vi "Datacluster remove duplicates_sort_test.vi"(5 "Remove duplicate":bool=TRUE, 6 "tolerance":dbl format="%.3e", 7 "ascending":bool=TRUE, 9 "Sort?":bool=TRUE) -> ()   [LabVIEW 2020]
panel:
  out "comparative":dbl
  out "output":dbl[][](array[numeric])=[[0.0, 0.0, -1.0], [1.0, 3.0, 4.0], [2.0, 0.0, 0.0], [3.0, 0.0, 0.0], [4.0, 1.0, 0.0], [6.0, 0.0, 5.0], [7.0, 0.0, 0.0], [8.0, 0.0, 0.0], [9.0, 0.0, 0.0]]
  in  "all rows":dbl[][](array[numeric])=[[7.0, 0.0, 0.0], [0.0, 0.0, -1.0], [2.0, 0.0, 0.0], [4.0, 1.0, 0.0], [6.0, 0.0, 5.0], [7.0, 0.0, 0.0], [0.0, 0.0, 0.0], [1.0, 3.0, 4.0], [9.0, 0.0, 0.0], [2.0, 0.0, 0.0], [3.0, 0.0, 0.0], [0.0, 0.0, 0.0], [2.0, 0.0, 0.0], [8.0, 0.0, 0.0]]
  in  "target column":u16
  # "(1) Data are sorted ascending or descending order.\n(2) Remove duplicate\n      i) Neighboring two data points are compared, if determined to be a duplicate, the second data point will be removed.\n      ii) Repeat i) unitl no duplicates found."
  # "Caution: All rows will be affected."
  # "(1) Select datasets to be processed"
  # "(2) Sort"
  # "i) Sort ?"
  # "ii) Ascending or descendingwhich order?"
  # "descending"
  # "(3) Remove duplicate? Tolerance?"
  # "(duplicate if \ndata difference <= (max-min) * tolerance"
  # "(4) Start processing"
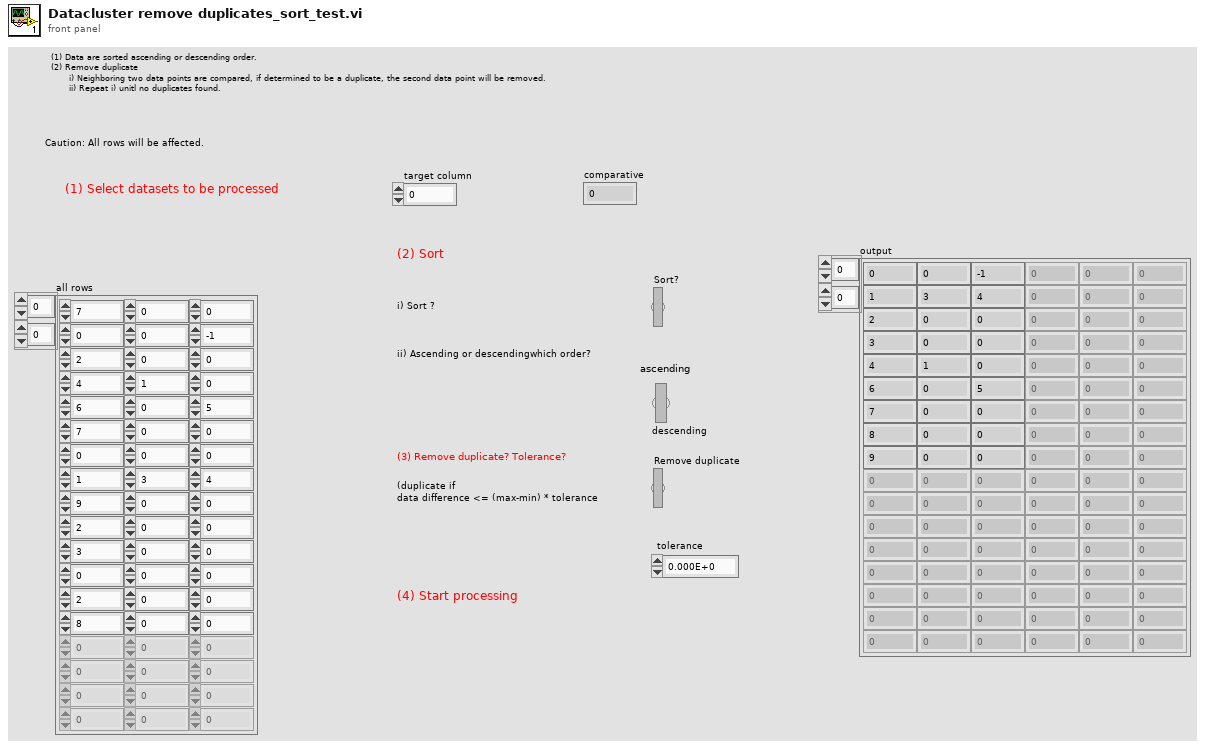
[diagram p1: front panel]
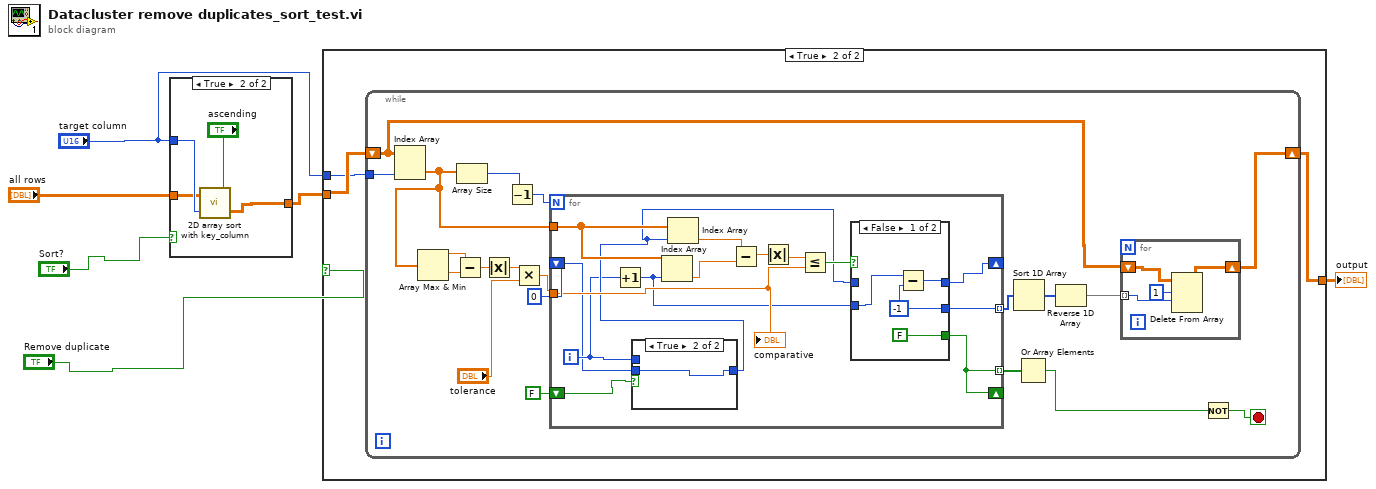
[diagram p0: block diagram]
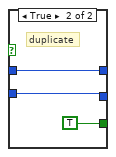
[diagram p4: hidden frame]
diagram:
  n1 = case shown="True" "Sort?" {
    tunnel: [w7 w11] -> w5
    tunnel: "target column" -> [_ w9]
    tunnel: "all rows" -> [w7 w8]
    frame False {
    }
    frame True {
      n2 = call "2D array sort with key_column.vi"("ascending"="ascending", "key column"=w9, "input"=w8) -> ("output"=w11:dbl[][])
    }
  }
  n3 = case shown="True" "Remove duplicate" {
    tunnel: [w12 w13] -> w2
    tunnel: w5 -> [w12 w15]
    tunnel: "target column" -> [_ w14]
    frame False {
    }
    frame True {
      n4 = while {
        tunnel: w14 -> [w29]
        shift-right: [w20] -> w13
        shift-left: w15 -> [w21]
        stop <- w30 stop-if-true
        n5 = Index Array(array=w21, index (col)=w29) -> (element=w24:dbl[])  [unwired: 1 in]
        n6 = Array Max & Min(array=w24) -> (max value=w23:dbl, min value=w25:dbl)  [unwired: 2 out]
        n7 = Subtract(x=w23, y=w25) -> (x-y=w26:dbl)
        n8 = Array Size(array=w24) -> (size(s)=w17:i32)
        n9 = Absolute Value(x=w26) -> (abs(x)=w28:dbl)
        n10 = Decrement(x=w17) -> (x-1=w16:i32)
        n11 = Multiply(x=w28, y="tolerance") -> (x*y=w22:dbl)
        n12 = for {
          N: w16 -> [_]
          tunnel: w24 -> [w54]
          tunnel: w22 -> [w50]
          tunnel: [w42] -> w34 mode=indexing
          tunnel: [w46] -> w32 mode=indexing
          shift-right: [w41] -> _
          shift-left: 0 -> [w40]
          shift-right: [w46] -> _
          shift-left: FALSE -> [w45]
          i -> [w43]
          n13 = Increment(x=w43) -> (x+1=w48:i32)
          n14 = case shown="True" w45 {
            tunnel: w43 -> [w55 _]
            tunnel: [w55 w56] -> w44
            tunnel: w40 -> [_ w56]
            frame False {
            }
            frame True {
            }
          }
          n15 = Index Array(array=w54, index=w48) -> (element=w53:dbl)
          n16 = Index Array(array=w54, index=w44) -> (element=w52:dbl)
          n17 = Subtract(x=w52, y=w53) -> (x-y=w51:dbl)
          n18 = Absolute Value(x=w51) -> (abs(x)=w47:dbl)
          n19 = Less Or Equal?(x=w47, y=w50) -> (x <= y?=w49:bool)
          n20 = case shown="False" w49 {
            tunnel: w48 -> [w58 w63]
            tunnel: [w57 w63] -> w42
            tunnel: [FALSE TRUE] -> w46
            tunnel: w44 -> [_ w61]
            tunnel: [w59 w61] -> w41
            frame False {
              w57 = -1
              n21 = Subtract(x=w58, y=w57) -> (x-y=w59:i32)
            }
            frame True {
              # "duplicate"
            }
          }
          "comparative" <- w50
        }
        n22 = Sort 1D Array(array=w34) -> (sorted array=w35:i32[])
        n23 = Or Array Elements(Boolean array=w32) -> (logical OR=w31:bool)
        n24 = Reverse 1D Array(array=w35) -> (reversed array=w33:i32[])
        n25 = for {
          tunnel: w33 -> [w38] mode=indexing
          shift-right: [w36] -> w20
          shift-left: w21 -> [w37]
          n26 = Delete From Array(array=w37, length=1, index (row)=w38) -> (array with subset deleted=w36:dbl[][])  [unwired: 1 in, 1 out]
        }
        n27 = Not(x=w31) -> (.not. x?=w30:bool)
      }
    }
  }
  "output" <- w2
